vi "Init.vi"(8 "error in (no error)":errorcluster, 11 "Server":refnum<class "Server.lvclass">) -> (0 "error out":errorcluster, 3 "Arguments out":refnum<class "Values.lvclass">)   [LabVIEW 2020, in "HTTP Server.lvlib" / "Values.lvclass"]
uses:
  Values.lvclass
  Server/Server.lvclass
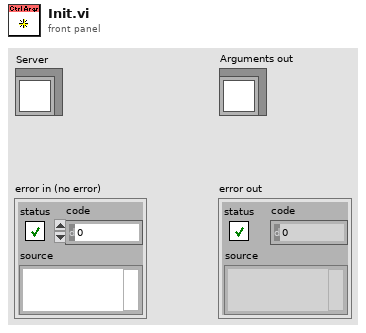
[diagram p1: front panel]
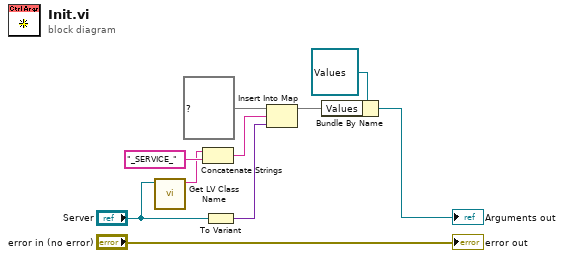
[diagram p0: block diagram]
diagram:
  n1 = call <vilib>:"Get LV Class Name.vi"("object"="Server") -> ("class name"=w8:string)  [unwired: 9 in, 1 out]
  n2 = Concatenate Strings(w8, "_SERVICE_" ("string")) -> (w3:string)
  n3 = To Variant(anything="Server") -> (Variant=w1:variant)
  n4 = Insert Into Map(map in=map{string, variant} {} ("Arguments"), key=w3, value=w1) -> (map out=w4:map{string, variant})  [unwired: 2 out]
  n5 = Bundle By Name(cluster=refnum<class "Values.lvclass"> refnum ("Arguments out"), "Values"=w4) -> (→"Arguments out":refnum<class "Values.lvclass">)
  "error out" <- "error in (no error)"
